vi "Configure Digital Output.vi"(0 "VISA resource name":refnum<visa-resource-name>, 1 "Autoclear Digital Output (F: Disable)":bool, 5 "Digital Output Bit Pattern (15)":u16=15, 9 "Autoclear Delay (1e-4 s)":dbl=0.0001, 11 "error in (no error)":errorcluster) -> (4 "VISA resource name out":refnum<visa-resource-name>, 15 "error out":errorcluster)   [LabVIEW 2021, in "Keithley 648X Series.lvlib"]
doc: "Configures the digital output that occurs after every binning operation. The digital output serves as a \"no action\" condition for the component handler. \n\n<b>Notes:</b>\n1)This VI is part of the component handler interfacing VIs.\n2)This supports model 6487 only"
uses:
  <instrlib>/Keithley 648X Series/Keithley 648X Series.lvlib
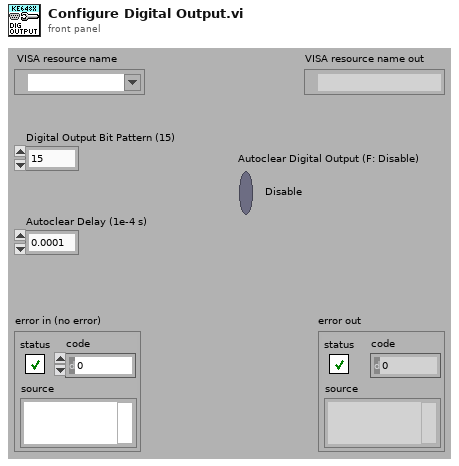
[diagram p1: front panel]
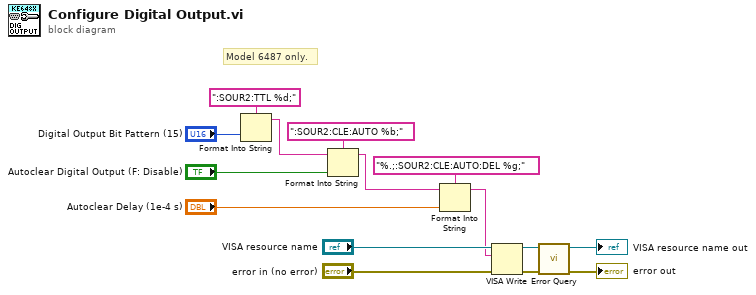
[diagram p0: block diagram]
diagram:
  # "Model 6487 only."
  n1 = Format Into String(format string=":SOUR2:TTL %d;", "Digital Output Bit Pattern (15)") -> (resulting string=w5:string)  [unwired: 2 in, 1 out]
  n2 = Format Into String(format string=":SOUR2:CLE:AUTO %b;", initial string=w5, "Autoclear Digital Output (F: Disable)") -> (resulting string=w4:string)  [unwired: 1 in, 1 out]
  n3 = Format Into String(format string="%.;:SOUR2:CLE:AUTO:DEL %g;", initial string=w4, "Autoclear Delay (1e-4 s)") -> (resulting string=w1:string)  [unwired: 1 in, 1 out]
  n4 = VISA Write(VISA resource name="VISA resource name", write buffer=w1, error in (no error)="error in (no error)") -> (VISA resource name out=w11:refnum<visa-resource-name>, error out=w10:errorcluster)  [unwired: 1 out]
  n5 = call <instrlib>:"Error Query.vi"("error in (no error)"=w10, "VISA resource name"=w11) -> ("error out"=→"error out":errorcluster, "VISA resource name out"=→"VISA resource name out":refnum<visa-resource-name>)  [unwired: 6 in, 2 out]
